vi "Channel Array Size Error Test.vi"(8 "error in (no error)":errorcluster, 11 "NI 9475 Test in":refnum<class "NI 9475 Test.lvclass">) -> (0 "error out":errorcluster, 3 "NI 9475 Test out":refnum<class "NI 9475 Test.lvclass">)   [LabVIEW 2019, in "NI 9475 Test.lvclass"]
uses:
  NI 9475 Test.lvclass
  Scripting/Modules/NI 9475/NI 9475.lvclass
  Module Test.lvclass
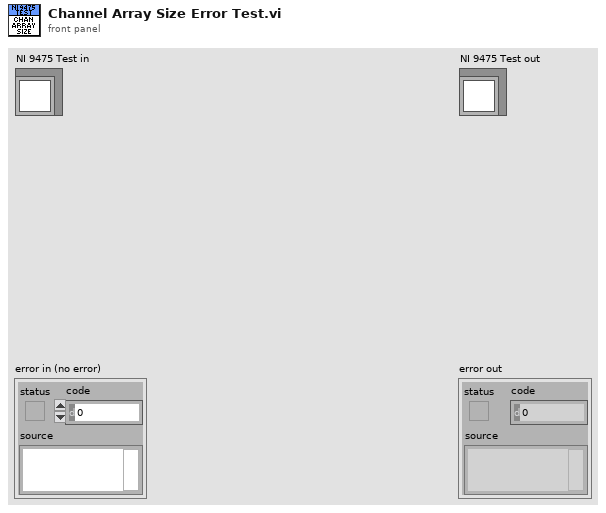
[diagram p1: front panel]
types:
  T1 = typedef "Scan Engine Scripting.lvlib/digital channel settings.ctl" = cluster{"name":string, "default value":bool}
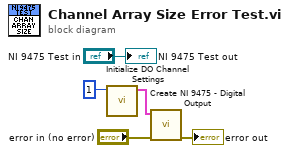
[diagram p0: block diagram]
diagram:
  n1 = call "Initialize DO Channel Settings.vi"("array size"=1) -> ("channel settings"=w4:T1[])  [unwired: 10 in]
  n2 = call "Create NI 9475 - Digital Output.vi"("error in"="error in (no error)", "channel settings"=w4) -> ("error out"=→"error out":errorcluster)  [unwired: 8 in, 1 out]
  "NI 9475 Test out" <- "NI 9475 Test in"
